vi "Set Guard Connection.vi"(8 "error in (no error)":errorcluster, 10 "Guard Connection (T: Internal)":bool=TRUE, 11 "VISA resource name":refnum<visa-resource-name>) -> (0 "error out":errorcluster, 3 "VISA resource name out":refnum<visa-resource-name>)   [LabVIEW 2011, in "Fluke 5XXX Series Multicalibrators.lvlib"]
doc: "This VI connects or disconnects the internal guard shield from the LO binding post.\n\nNote:\n\nThis VI is available only for instrument models 5520A, 5700A, 5720A and 57LFC."
uses:
  Fluke 5XXX Series Multicalibrators.lvlib
panel:
  # "Internal"
  # "External"
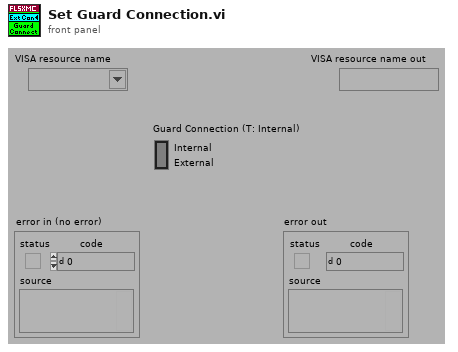
[diagram p1: front panel]
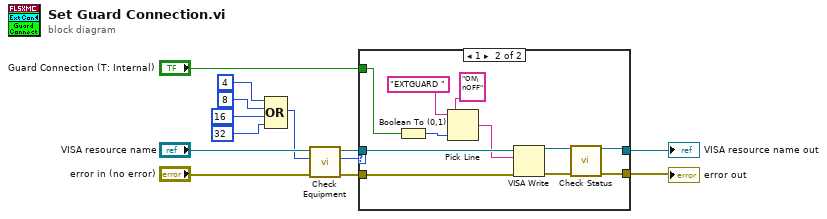
[diagram p0: block diagram]
diagram:
  n1 = Compound Arithmetic op=OR(4 ("Numeric"), 8 ("Numeric"), 16 ("Numeric"), 32 ("Numeric")) -> (w2:i32)
  n2 = call "Check Equipment.vi"("error in (no error)"="error in (no error)", "Bit Mask"=w2, "VISA resource name"="VISA resource name") -> ("error out"=w13:errorcluster, "Present?"=w12:u32, "VISA resource name out"=w11:refnum<visa-resource-name>)  [unwired: 6 in]
  n3 = case shown="1" w12 {
    tunnel: "Guard Connection (T: Internal)" -> [_ w23]
    tunnel: [w14 w18] -> w6
    tunnel: w13 -> [w15 w22]
    tunnel: w11 -> [w14 w21]
    tunnel: [w15 w19] -> w7
    frame 0, Default {
    }
    frame 1 {
      n4 = Boolean To (0,1)(Boolean=w23) -> (0, 1=w24:i16)
      n5 = Pick Line(string ("")="EXTGUARD " ("Reset Command"), multi-line string="ON\nOFF", line index=w24) -> (output string=w20:string)
      n6 = VISA Write(VISA resource name=w21, write buffer=w20, error in (no error)=w22) -> (VISA resource name out=w17:refnum<visa-resource-name>, error out=w16:errorcluster)  [unwired: 1 out]
      n7 = call "Check Status.vi"("VISA resource name"=w17, "error in (no error)"=w16) -> ("VISA resource name out"=w18:refnum<visa-resource-name>, "error out"=w19:errorcluster)  [unwired: 12 in]
    }
  }
  "VISA resource name out" <- w6
  "error out" <- w7
